vi "Setup Retaining Channel.vi"(4 "Excluded (None)":refnum<class "Message.lvclass">[](array[class]), 6 "Included (All)":refnum<class "Message.lvclass">[](array[class]), 7 "Emit Status Messages (F)":bool, 8 "error in (no error)":errorcluster, 11 "Pub Sub Retaining Message Channel in":refnum<class "Pub Sub Retaining Message Channel.lvclass">) -> (0 "error out":errorcluster, 3 "Pub Sub Retaining Message Channel out":refnum<class "Pub Sub Retaining Message Channel.lvclass">)   [LabVIEW 2020, in "Actor Pub Sub Channels.lvlib" / "Pub Sub Retaining Message Channel.lvclass"]
uses:
  Pub Sub Retaining Message Channel.lvclass
  Pub Sub Retaining Message Channel.lvclass/Pub Sub Retaining Message Channel.ctl
  Pub Sub Message Channel/Pub Sub Message Channel.lvclass
  C:/Users/Simon/Documents/GitHub/LV-Actor-Pub-Sub/Source/Actor Pub Sub Channels/Pub Sub Message Channel/Pub Sub Message Channel.lvclass
  C:/Users/Simon/Documents/GitHub/LV-Actor-Pub-Sub/Source/Actor Pub Sub Channels/Pub Sub Retaining Message Channel/Pub Sub Retaining Message Channel.lvclass
  <vilib>/ActorFramework/Message/Message.lvclass
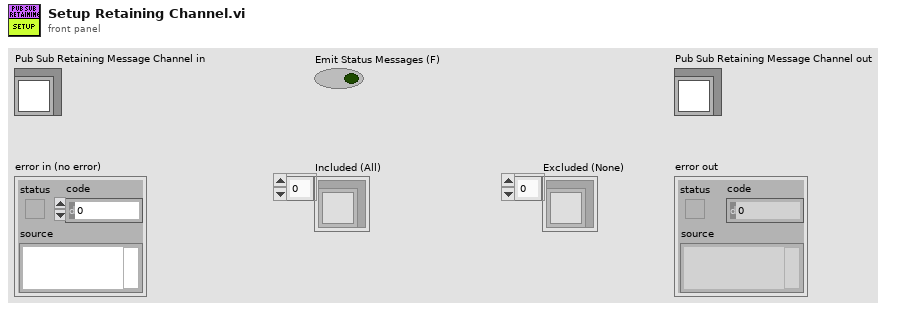
[diagram p1: front panel]
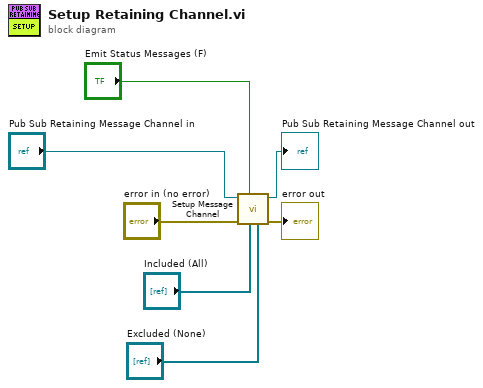
[diagram p0: block diagram]
diagram:
  n1 = call "Setup Message Channel.vi"("Excluded (None)"="Excluded (None)", "Included (All)"="Included (All)", "Emit Status Messages (F)"="Emit Status Messages (F)", "error in (no error)"="error in (no error)", "Pub Sub Message Channel in"="Pub Sub Retaining Message Channel in") -> ("error out"=→"error out":errorcluster, "Pub Sub Message Channel out"=→"Pub Sub Retaining Message Channel out":refnum<class "Pub Sub Retaining Message Channel.lvclass">)  [unwired: 5 in]
